vi "GCMPlugin_GetInterfacePath.vi"(8 "error in (no error)":errorcluster, 11 "_BasicVIDocumentation in":refnum<class "BasicClassDocumentation.lvclass">) -> (0 "error out":errorcluster, 2 "Path":path, 3 "_BasicVIDocumentation out":refnum<class "BasicClassDocumentation.lvclass">)   [LabVIEW 2014, in "BasicClassDocumentation.lvlib" / "BasicClassDocumentation.lvclass"]
uses:
  BasicClassDocumentation.lvclass
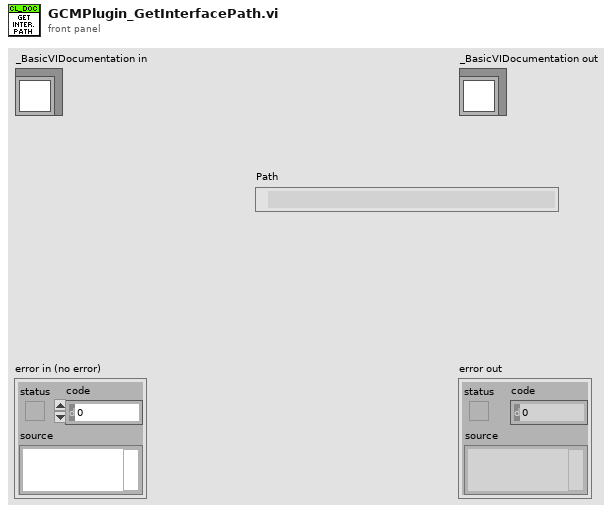
[diagram p1: front panel]
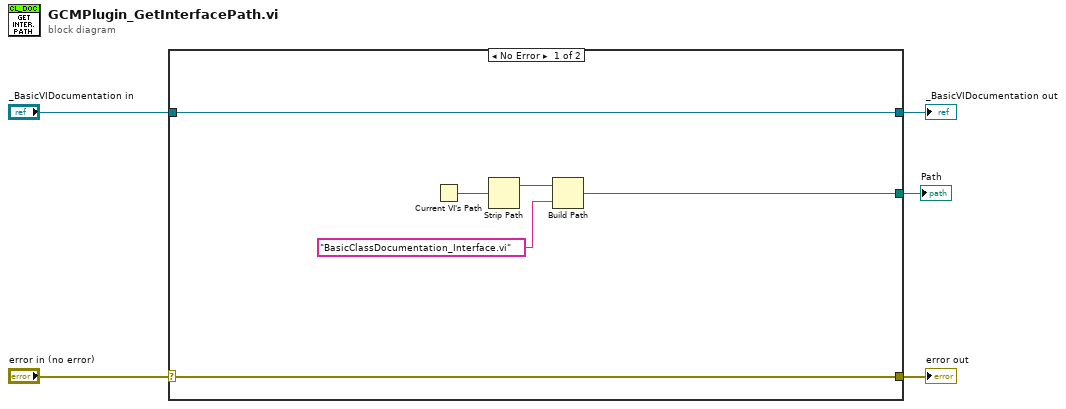
[diagram p0: block diagram]
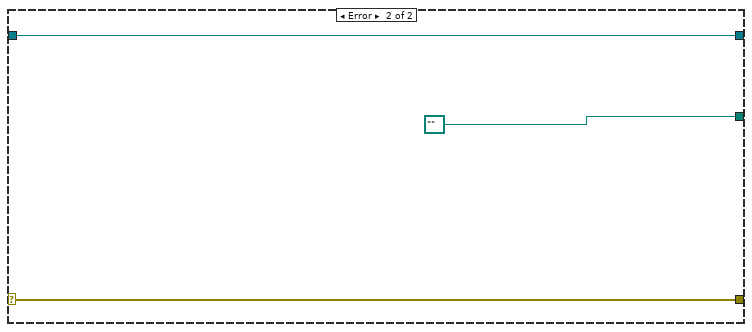
[diagram p2: hidden frame]
diagram:
  n1 = case shown="No Error" "error in (no error)" {
    selector: "error in (no error)" -> [w10 w14]
    tunnel: [w10 w14] -> w4
    tunnel: [w11 w13] -> w2
    tunnel: "_BasicVIDocumentation in" -> [w11 w13]
    tunnel: [w6 path "" ("Path")] -> w1
    frame No Error {
      n2 = Current VI's Path() -> (path=w9:path)
      n3 = Strip Path(path=w9) -> (stripped path=w8:path)  [unwired: 1 out]
      n4 = Build Path(base path=w8, name or relative path="BasicClassDocumentation_Interface.vi") -> (appended path=w6:path)
    }
    frame Error {
    }
  }
  "error out" <- w4
  "_BasicVIDocumentation out" <- w2
  "Path" <- w1
